vi "Write State.vi"(8 "error in":errorcluster, 10 "State":T1=enum."Idle", 11 "Base Software in":refnum<class "Base Software.lvclass">) -> (0 "error out":errorcluster, 3 "Base Software out":refnum<class "Base Software.lvclass">)   [LabVIEW 2019, in "Base Software.lvlib" / "Main.lvlib" / "Base Software.lvclass"]
uses:
  Project/Base Software.lvclass
  builds/Engine/Engine.lvlibp/Custom Controls/System Status.ctl
  Project/Base Software.lvclass/Base Software.ctl
  builds/Engine/Engine.lvlibp/Project/Engine.lvclass
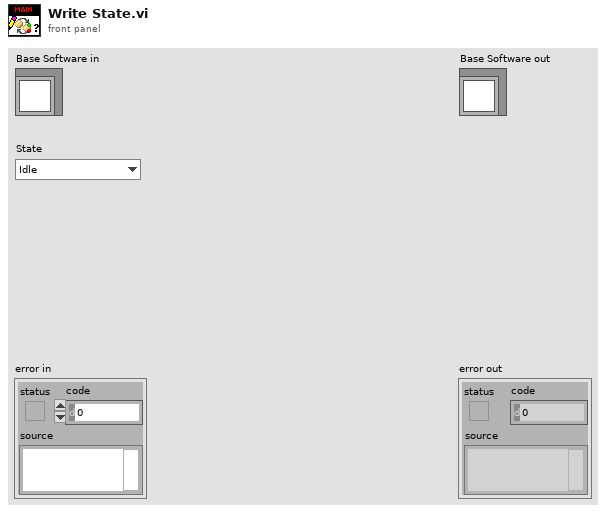
[diagram p1: front panel]
types:
  T1 = typedef "Engine.lvlibp/Engine.lvclass/System Status.ctl" = enum16{"Logged Off", "UUT_Info_Missing", "Idle", "Error", "Warning", "Loading", "Config", "Manual", "Automation", "Report_View", "Previous"}
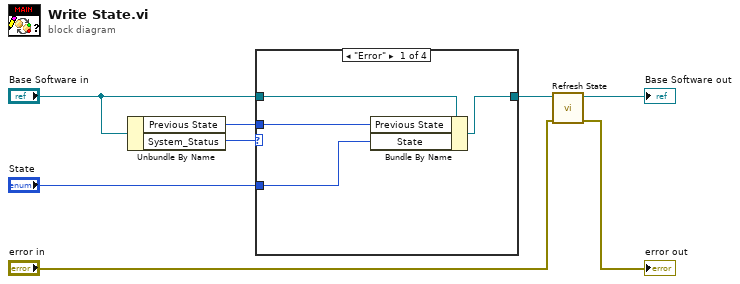
[diagram p0: block diagram]
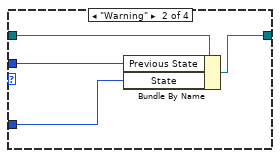
[diagram p2: hidden frame]
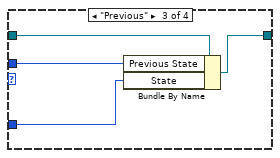
[diagram p3: hidden frame]
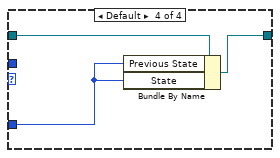
[diagram p4: hidden frame]
diagram:
  n1 = Unbundle By Name("Base Software in") -> ("Previous State"=w6:T1, "System_Status"=w8:T1)
  n2 = case shown="\"Error\"" w8 {
    tunnel: "Base Software in" -> [w12 w16 w20 w23]
    tunnel: w6 -> [w10 w14 w17 _]
    tunnel: [w11 w15 w19 w22] -> w4
    tunnel: "State" -> [w9 w13 w18 w21]
    frame "Error" {
      n3 = Bundle By Name(cluster=w12, "Previous State"=w10, "State"=w9) -> (w11:refnum<class "Base Software.lvclass">)
    }
    frame "Warning" {
      n4 = Bundle By Name(cluster=w16, "Previous State"=w14, "State"=w13) -> (w15:refnum<class "Base Software.lvclass">)
    }
    frame "Previous" {
      n5 = Bundle By Name(cluster=w20, "Previous State"=w17, "State"=w18) -> (w19:refnum<class "Base Software.lvclass">)
    }
    frame Default {
      n6 = Bundle By Name(cluster=w23, "Previous State"=w21, "State"=w21) -> (w22:refnum<class "Base Software.lvclass">)
    }
  }
  n7 = call "Refresh State.vi"("error in"="error in", "Base Software in"=w4) -> ("error out"=→"error out":errorcluster, "Base Software out"=→"Base Software out":refnum<class "Base Software.lvclass">)  [unwired: 8 in]
